vi "Unbundle and Calc Grating.vi"(8 "error in (no error)":errorcluster, 9 "SLM Params":T2 {"Centre X" format="%.3g"; "Centre Y" format="%.3g"}, 10 "Spot Settings":T1, 11 "holo_init":u8[](array[numeric])) -> (0 "error out":errorcluster, 3 "Grating Holo":u8[](array[numeric]))   [LabVIEW 2020]
uses:
  _controls/PCIe SLM params.ctl
  <userlib>/SLM ImageGen/SLM ImageGen.lvlib
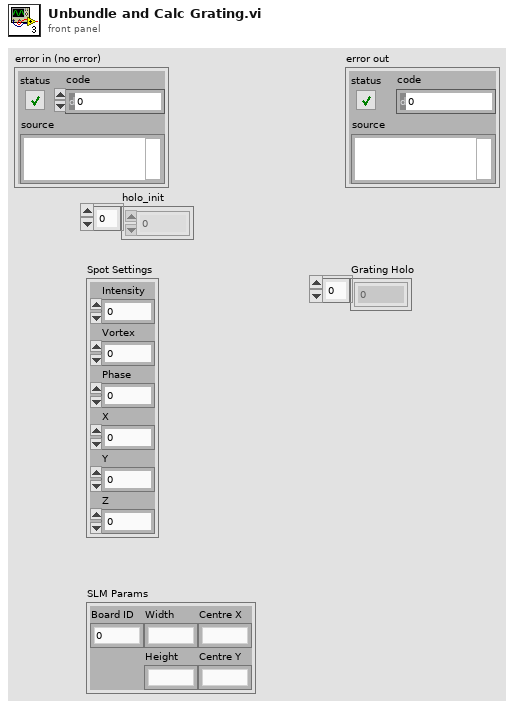
[diagram p1: front panel]
types:
  T1 = cluster{"Intensity":dbl, "Vortex":dbl, "Phase":dbl, "X":dbl, "Y":dbl, "Z":dbl}
  T2 = typedef "PCIe SLM params.ctl" = cluster{"Width":dbl, "Height":dbl, "Board ID":i32, "Centre Y":dbl, "Centre X":dbl}
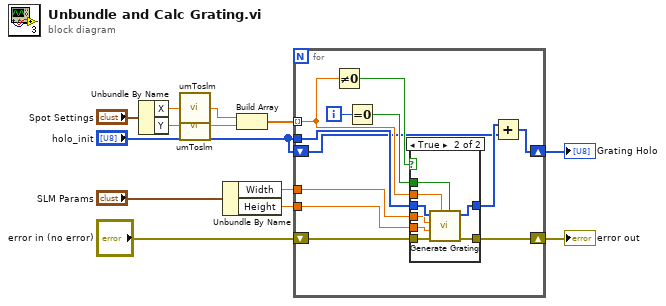
[diagram p0: block diagram]
diagram:
  n1 = Unbundle By Name("Spot Settings") -> ("X"=w7:dbl, "Y"=w4:dbl)
  n2 = call "umToslm.vi"("X (um)"=w7) -> ("SLM Period"=w6:dbl)
  n3 = call "umToslm.vi"("X (um)"=w4) -> ("SLM Period"=w3:dbl)
  n4 = Unbundle By Name("SLM Params") -> ("Width"=w12:dbl, "Height"=w13:dbl)
  n5 = Build Array(w6, w3) -> (w10:dbl[])
  n6 = for {
    tunnel: w10 -> [w24] mode=indexing
    tunnel: "holo_init" -> [w25]
    tunnel: w12 -> [w20]
    tunnel: w13 -> [w19]
    shift-right: [w18] -> w5
    shift-left: "holo_init" -> [w16]
    shift-right: [w15] -> w2
    shift-left: "error in (no error)" -> [w14]
    i -> [w22]
    n7 = Not Equal To 0?(x=w24) -> (x != 0?=w23:bool)
    n8 = Equal To 0?(x=w22) -> (x = 0?=w21:bool)
    n9 = case shown="True" w23 {
      tunnel: w25 -> [w27 w35]
      tunnel: w19 -> [_ w33]
      tunnel: w20 -> [_ w32]
      tunnel: [w27 w34] -> w17
      tunnel: w24 -> [_ w31]
      tunnel: w21 -> [_ w30]
      tunnel: [w26 w29] -> w15
      tunnel: w14 -> [w26 w28]
      frame False {
      }
      frame True {
        n10 = call <userlib>:"Generate Grating.vi"("horizontal"=w30, "Period"=w31, "error in (no error)"=w28, "height"=w33, "width"=w32, "holoBuffer"=w35) -> ("error out"=w29:errorcluster, "Grating holo"=w34:u8[])  [unwired: 4 in]
      }
    }
    n11 = Add(x=w17, y=w16) -> (x+y=w18:u8[])
  }
  "Grating Holo" <- w5
  "error out" <- w2
